vi "Message_Reconstructor.vi"(9 "Wp2":u8[](array[numeric]), 10 "Wp1":u8[](array[numeric]), 11 "Wc":u8[](array[numeric])) -> (2 "W2":u8[](array[numeric]), 3 "W1":u8[](array[numeric]))   [LabVIEW 2022 SP3]
panel:
  in  "No. Common Bits":i32=3
  in  "No. Total Bits":i32=6
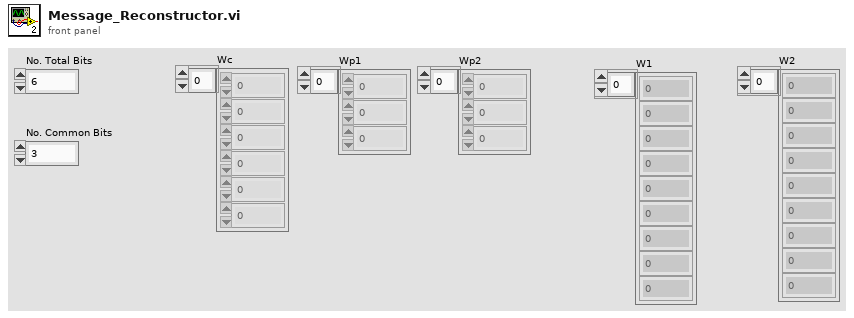
[diagram p1: front panel]
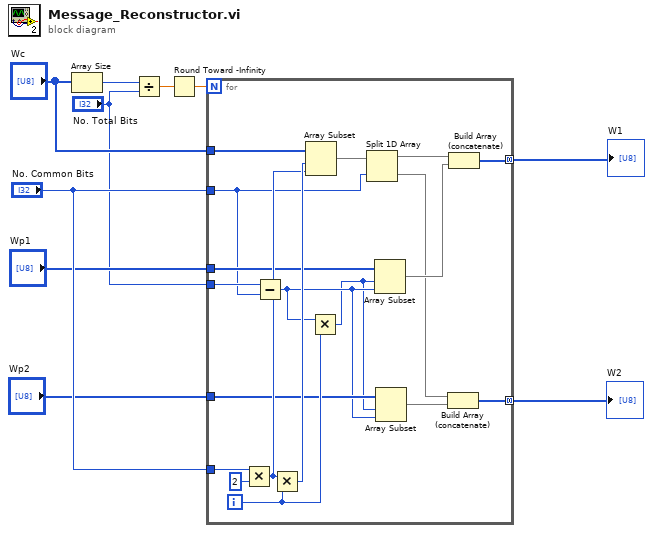
[diagram p0: block diagram]
diagram:
  n1 = Array Size(array="Wc") -> (size(s)=w10:i32)
  n2 = Divide(x=w10, y="No. Total Bits") -> (x/y=w9:dbl)
  n3 = Round Toward -Infinity(1:w9) -> (0:w8:dbl)
  n4 = for {
    N: w8 -> [_]
    tunnel: "Wc" -> [w29]
    tunnel: "No. Common Bits" -> [w27]
    tunnel: "No. Common Bits" -> [w21]
    tunnel: [w17] -> w5 mode=concatenating
    tunnel: [w11] -> w4 mode=concatenating
    tunnel: "Wp1" -> [w23]
    tunnel: "No. Total Bits" -> [w22]
    tunnel: "Wp2" -> [w16]
    i -> [w20]
    n5 = Multiply(x=w27, y=u8 2) -> (x*y=w25:i32)
    n6 = Subtract(x=w22, y=w21) -> (x-y=w15:i32)
    n7 = Multiply(x=w25, y=w20) -> (x*y=w26:i32)
    n8 = Array Subset(array=w29, index=w26, length=w25) -> (w24:u8[])
    n9 = Multiply(x=w15, y=w20) -> (x*y=w14:i32)
    n10 = Split 1D Array(array=w24, index=w21) -> (first subarray=w19:u8[], second subarray=w13:u8[])
    n11 = Array Subset(array=w23, index=w14, length=w15) -> (w18:u8[])
    n12 = Array Subset(array=w16, index=w14, length=w15) -> (w12:u8[])
    n13 = Build Array (concatenate)(w13, w12) -> (w11:u8[])
    n14 = Build Array (concatenate)(w19, w18) -> (w17:u8[])
  }
  "W1" <- w5
  "W2" <- w4
